vi "Write Comp Motors with Brake Config.vi"(8 "error in (no error)":errorcluster, 10 "Comp Motors with Brake Config":T1={"Brake Channel"=enum."Solenoid 6", "Pneumatics CAN ID"=3}, 11 "Comp Motors with Brake in":refnum<class "Comp Motors with Brake.lvclass">) -> (0 "error out":errorcluster, 3 "Comp Motors with Brake out":refnum<class "Comp Motors with Brake.lvclass">)   [LabVIEW 2014, in "Comp Motors with Brake.lvlib" / "Comp Motors with Brake.lvclass"]
uses:
  Comp Motors with Brake.lvclass
  Comp Motors with Brake Config.ctl
  <vilib>/Rock Robotics/WPI/Solenoid/WPI_SolenoidChannel.ctl
  Comp Motors with Brake.lvclass/Comp Motors with Brake.ctl
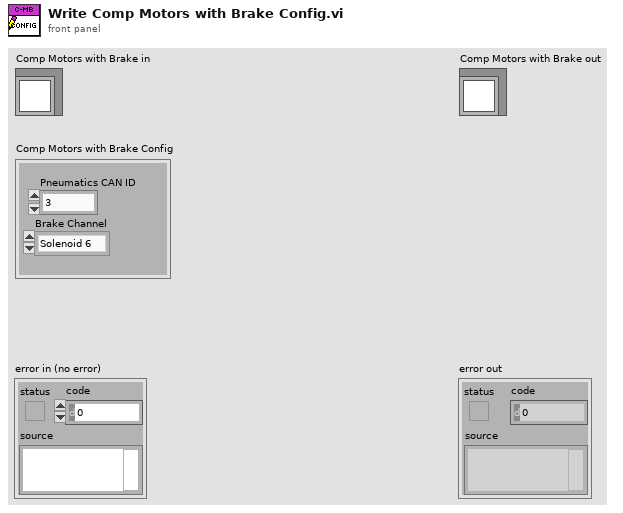
[diagram p1: front panel]
types:
  T1 = typedef "Comp Motors with Brake.lvlib/Comp Motors with Brake.lvclass/Comp Motors with Brake Config.ctl" = cluster{"Brake Channel":T2, "Pneumatics CAN ID":u8}
  T2 = typedef "WPI_SolenoidChannel.ctl" = enum8{"Solenoid 0", "Solenoid 1", "Solenoid 2", "Solenoid 3", "Solenoid 4", "Solenoid 5", "Solenoid 6", "Solenoid 7", "Invalid"}
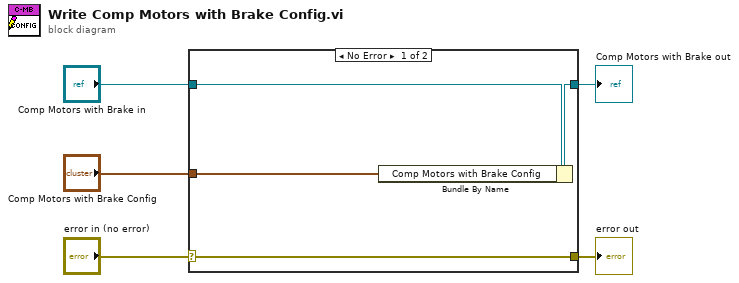
[diagram p0: block diagram]
diagram:
  n1 = case shown="No Error" "error in (no error)" {
    selector: "error in (no error)" -> [w9 w10]
    tunnel: [w9 w10] -> w4
    tunnel: [w7 w11] -> w2
    tunnel: "Comp Motors with Brake in" -> [w8 w11]
    tunnel: "Comp Motors with Brake Config" -> [w6 _]
    frame No Error {
      n2 = Bundle By Name(cluster=w8, "Comp Motors with Brake Config"=w6) -> (w7:refnum<class "Comp Motors with Brake.lvclass">)
    }
    frame Error {
    }
  }
  "error out" <- w4
  "Comp Motors with Brake out" <- w2
